vi "Main.vi"() -> ()   [LabVIEW 2019]
doc: "The myRIO Project template acquires acceleration data from the onboard accelerometer and displays the changes of acceleration values in a waveform chart."
uses:
  <vilib>/myRIO/Instrument Drivers/Onboard IO/UART/typedef/VISA Configuration.ctl
  <vilib>/myRIO/Common/Instrument Driver Framework/myRIO v1.0/UART/vis/myRIO v1.0 Close UART.vi
  <vilib>/FPGAPlugInAG/myRIO-1900/niLvFpga_Open_myRIO-1900.vi
  <vilib>/rvi/interface/common/dynamic/niFpgaDynamicAddResources.vi
  <vilib>/Instr/_visa.llb/VISA Configure Serial Port (Instr).vi
  <vilib>/Utility/error.llb/Error Cluster From Error Code.vi
  <vilib>/rvi/errors/niLvFpgaAdjustHostInterfaceError.vi
  <vilib>/myRIO/Common/Instrument Driver Framework/Utilities/vis/FPGA Ref Manager.vi
  <vilib>/myRIO/Common/Instrument Driver Framework/myRIO v1.0/myRIO v1.0 Reset FPGA.vi
  <vilib>/myRIO/Common/Instrument Driver Framework/myRIO v1.0/IRQ/vis/myRIO v1.0 IRQ Info FGV.vi
  <vilib>/myRIO/Common/Instrument Driver Framework/myRIO v1.0/IRQ/vis/myRIO v1.0 Timer IRQ Info FGV.vi
  <vilib>/myRIO/Common/Instrument Driver Framework/myRIO v1.0/IRQ/vis/myRIO v1.0 ISR Agent.vi
  <vilib>/myRIO/Instrument Drivers/Utilities/vis/Reset Index.vi
  <vilib>/myRIO/Common/Instrument Driver Framework/myRIO v1.0/Resource Manager/vis/myRIO v1.0 Block Write Resource Manager.vi
  <vilib>/FPGAPlugInAG/Dynamic/niLvFpga_Close_Dynamic.vi
  <vilib>/rvi/interface/nirviOpenFPGA/nirviOpenFPGA.xnode
  FPGA Bitfiles/PickleRio_FPGATarget_StepperFPGA2.0_025pYRGnFXk.lvbitx
  SubVI/Stepper FPGA 2.0.vi
  <vilib>/myRIO/Express VI/Onboard IO/UART/UART Express VI.xnode
  <vilib>/rvi/interface/nirviReadWriteControl/nirviReadWriteControl.xnode
  <vilib>/rvi/interface/nirviCloseFPGA/nirviCloseFPGA.xnode
  <vilib>/myRIO/Instrument Drivers/Utilities/Utilities.lvlib
  NiFpgaLv.dll
  <vilib>/rvi/interface/Simulation/niFpgaSimulationCallBeginRW.vi
  <vilib>/myRIO/Instrument Drivers/Onboard IO/UART/UART.lvlib
panel:
  in  "KinematicArray":string[](array[string])
  out "Waveform Chart":dynamicdata(graph)
  in  "Speed Robot":dbl
  in  "Stop":bool
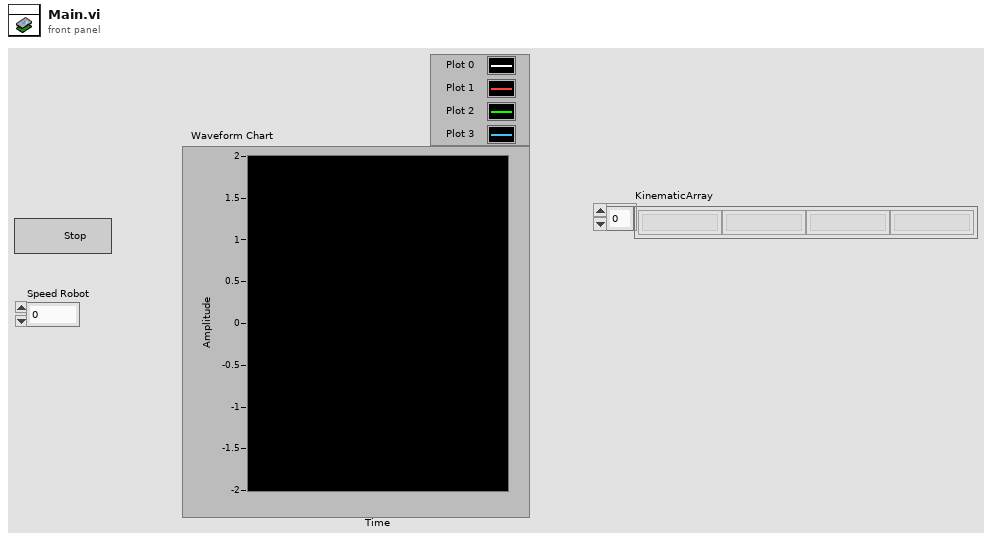
[diagram p1: front panel]
types:
  T1 = cluster{"proportional gain (Kc)":dbl, "integral time (Ti, min)":dbl, "derivative time (Td, min)":dbl}
  T2 = typedef "UART.lvlib/VISA Configuration.ctl" = cluster{"baud rate (9600)":u32, "data bits (8)":u16, "parity (0:none)":enum16{"None", "Odd", "Even", "Mark", "Space"}, "stop bits (10: 1 bit)":u16, "flow control (0:none)":u16, "termination char\n(0xA = '\\n' = LF) ":u8, "Enable Termination\nChar (T)":bool, "timeout (10sec)":u32}
  T3 = cluster{"L1":dbl, "L 2":dbl, "L 3":dbl, " s":dbl, "L1":dbl, "L 2":dbl, "L 3":dbl, " s":dbl}
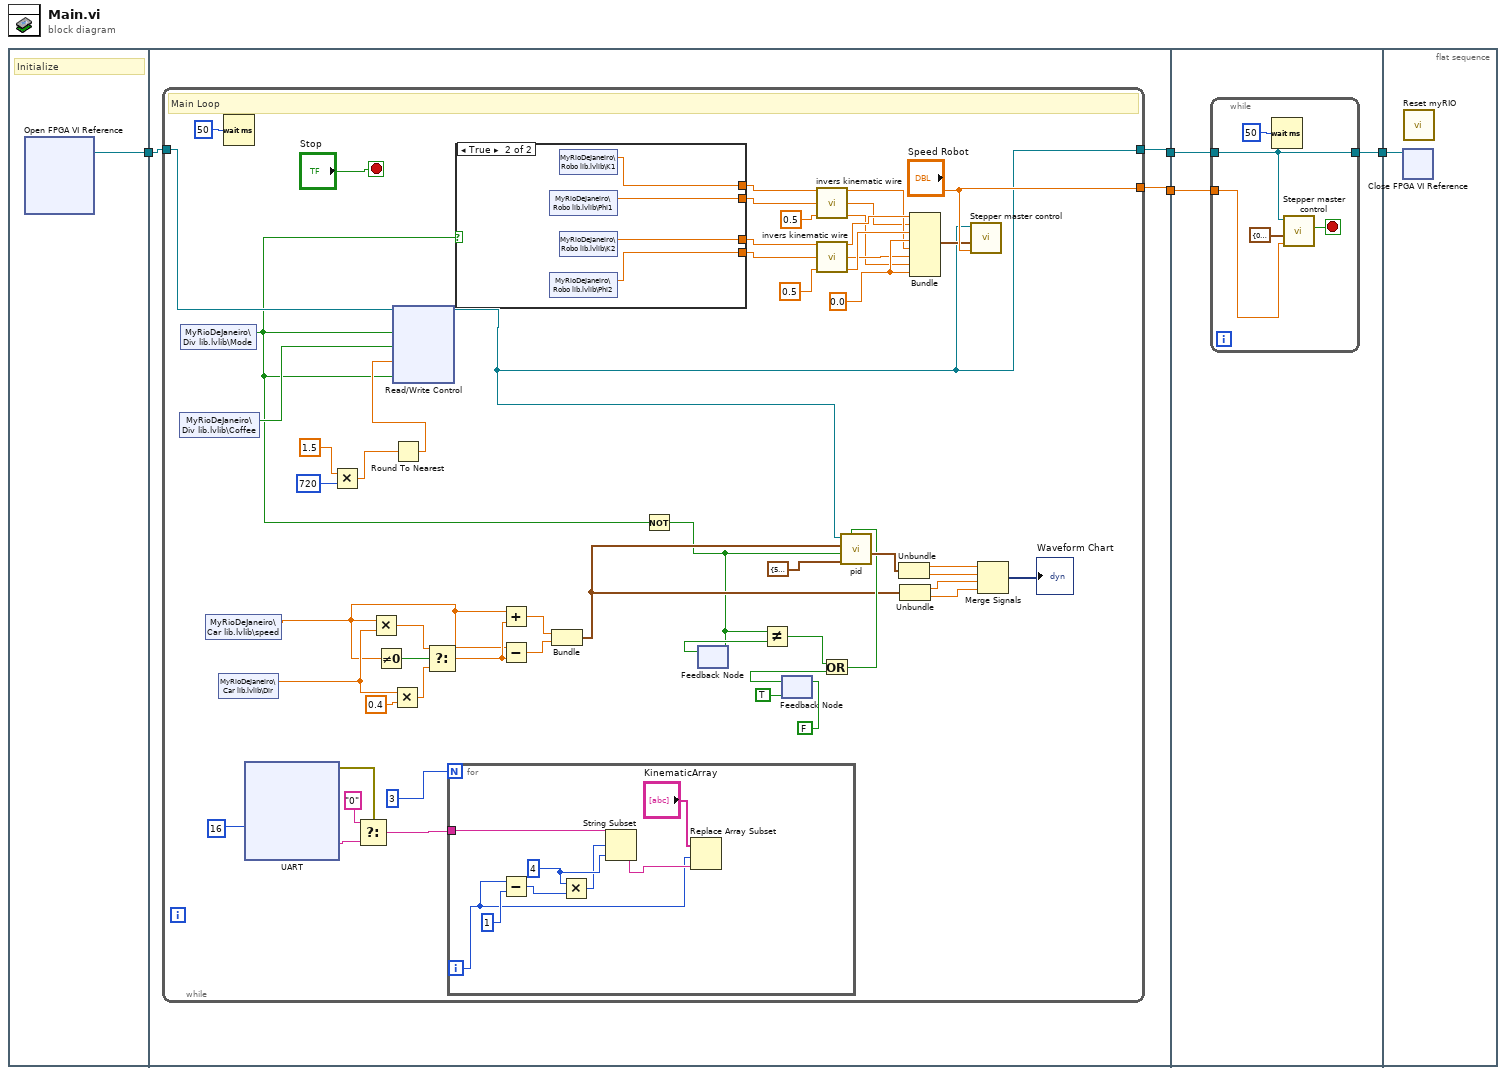
[diagram p0: block diagram]
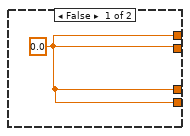
[diagram p2: hidden frame]
diagram:
  n1 = flat-sequence {
    tunnel: [w5] -> w4
    tunnel: w4 -> [w8]
    tunnel: [w7] -> w3
    tunnel: [w6] -> w2
    tunnel: w3 -> [w95]
    tunnel: w2 -> [w94]
    tunnel: [w93] -> w1
    tunnel: w1 -> [w101]
    frame #0 {
      # "Initialize"
      n2 = xnode "Open FPGA VI Reference"() -> ("FPGA VI Reference Out"=w5:refnum<k20>)  [unwired: 2 in, 1 out]
    }
    frame #1 {
      n3 = while {
        tunnel: w8 -> [w45]
        tunnel: ["Speed Robot"] -> w7
        tunnel: [w15] -> w6
        stop <- "Stop" stop-if-true
        w57 = 0.0 ("s")
        # "Main Loop"
        n4 = shared-variable "MyRioDeJaneiro\\Div lib.lvlib\\Coffee"() -> (w21:bool)  [unwired: 1 in, 1 out]
        n5 = shared-variable "MyRioDeJaneiro\\Div lib.lvlib\\Mode"() -> (w17:bool)  [unwired: 1 in, 1 out]
        n6 = shared-variable "MyRioDeJaneiro\\Car lib.lvlib\\speed"() -> (w23:dbl)  [unwired: 1 in, 1 out]
        n7 = shared-variable "MyRioDeJaneiro\\Car lib.lvlib\\Dir"() -> (w24:dbl)  [unwired: 1 in, 1 out]
        n8 = Wait (ms)(milliseconds to wait=u32 50) -> ()  [unwired: 1 out]
        n9 = xnode "UART"("Character Count"=16) -> ("Characters Read"=w13:string, "error out"=w12:errorcluster)  [unwired: 1 in]
        n10 = Multiply(x=1.5, y=i16 720) -> (x*y=w47:dbl)
        n11 = Select(t="0", s=w12, f=w13) -> (s? t:f=w11:string)
        n12 = Multiply(x=w23, y=w24) -> (x*y=w28:dbl)
        n13 = Not Equal To 0?(x=w23) -> (x != 0?=w29:bool)
        n14 = Multiply(x=w24, y=0.4 ("f")) -> (x*y=w26:dbl)
        n15 = Round To Nearest(number=w47) -> (nearest integer value=w46:dbl)
        n16 = xnode "Read/Write Control"("FPGA VI Reference In"=w45, "Pump"=w17, "Coffee"=w21, "cup size"=w46, "Boolean"=w17) -> ("FPGA VI Reference Out"=w15:refnum<k20>)  [unwired: 1 in, 1 out]
        n17 = Select(t=w28, s=w29, f=w26) -> (s? t:f=w27:dbl)
        n18 = for {
          N: 3 -> [_]
          tunnel: w11 -> [w71]
          i -> [w64]
          w68 = 4 ("y")
          n19 = Subtract(x=w64, y=1) -> (x-y=w69:i32)
          n20 = Multiply(x=w68, y=w69) -> (x*y=w67:i32)
          n21 = String Subset(string=w71, offset (0)=w67, length (rest)=w68) -> (substring=w66:string)
          n22 = Replace Array Subset(array="KinematicArray", new element=w66, index=w64) -> ()  [unwired: 1 out]
        }
        n23 = case shown="True" w17 {
          tunnel: [w88 w92] -> w16
          tunnel: [w88 w91] -> w50
          tunnel: [w88 w90] -> w49
          tunnel: [w88 w89] -> w18
          frame False {
            w88 = 0.0
          }
          frame True {
            n24 = shared-variable "MyRioDeJaneiro\\Robo lib.lvlib\\Phi1"() -> (w91:dbl)  [unwired: 1 in, 1 out]
            n25 = shared-variable "MyRioDeJaneiro\\Robo lib.lvlib\\Phi2"() -> (w89:dbl)  [unwired: 1 in, 1 out]
            n26 = shared-variable "MyRioDeJaneiro\\Robo lib.lvlib\\K1"() -> (w92:dbl)  [unwired: 1 in, 1 out]
            n27 = shared-variable "MyRioDeJaneiro\\Robo lib.lvlib\\K2"() -> (w90:dbl)  [unwired: 1 in, 1 out]
          }
        }
        n28 = Add(x=w23, y=w27) -> (x+y=w31:dbl)
        n29 = Subtract(x=w23, y=w27) -> (x-y=w30:dbl)
        n30 = Bundle(w31, w30) -> (w32:cluster{dbl, dbl})  [unwired: 1 in]
        n31 = Not(x=w17) -> (.not. x?=w20:bool)
        n32 = feedback-in #1(w20) -> ()
        n33 = feedback #1() -> (w43:bool)  [unwired: 1 in]
        n34 = Not Equal?(x=w20, y=w43) -> (x != y?=w42:bool)
        n35 = feedback #2(TRUE) -> (w41:bool)
        n36 = feedback-in #2(FALSE) -> ()
        n37 = call "invers kinematic wire.vi"("K"=w16, "phi"=w50, "s"=0.5) -> ("L1"=w53:dbl, "L 2"=w51:dbl, "L 3"=w52:dbl)  [unwired: 10 in]
        n38 = call "invers kinematic wire.vi"("K"=w49, "phi"=w18, "s"=0.5) -> ("L1"=w56:dbl, "L 2"=w54:dbl, "L 3"=w55:dbl)  [unwired: 10 in]
        n39 = Or(x=w42, y=w41) -> (x .or. y?=w33:bool)
        n40 = call "pid.vi"("reset"=w33, "PID gains"=T1 {"proportional gain (Kc)"=53.1, "integral time (Ti, min)"=0.003472, "derivative time (Td, min)"=0.0}, "Enable motors"=w20, "Speed"=w32, "Refnum in"=w15) -> ("output Speed"=w38:cluster{dbl, dbl})  [unwired: 4 in, 2 out]
        n41 = Unbundle(w38) -> (w35:dbl, w34:dbl)
        n42 = Unbundle(w32) -> (w37:dbl, w36:dbl)
        n43 = Bundle("L1"=w56, "L 2"=w51, "L 3"=w55, "s"=w57, "L1"=w53, "L 2"=w54, "L 3"=w52, "s"=w57) -> (w60:T3)  [unwired: 1 in]
        n44 = call "Stepper master control.vi"("Speed"="Speed Robot", "Pos"=w60, "FPGA VI Reference In"=w15) -> ()  [unwired: 8 in, 1 out]
        n45 = Merge Signals(w35, w34, w37, w36) -> (→"Waveform Chart":dynamicdata)
      }
    }
    frame #2 {
      n46 = while {
        tunnel: w95 -> [w99]
        tunnel: w94 -> [w96]
        tunnel: [w96] -> w93
        stop <- w97 stop-if-true
        n47 = Wait (ms)(milliseconds to wait=u32 50) -> ()  [unwired: 1 out]
        n48 = call "Stepper master control.vi"("Speed"=w99, "Pos"=cluster{dbl, dbl, dbl, dbl, dbl, dbl, dbl, dbl} {0.0, 0.0, 0.0, 0.0, 0.0, 0.0, 0.0, 0.0}, "FPGA VI Reference In"=w96) -> ("0?"=w97:bool)  [unwired: 8 in]
      }
    }
    frame #3 {
      n49 = xnode "Close FPGA VI Reference"("FPGA VI Reference In"=w101) -> ()  [unwired: 1 in, 1 out]
      n50 = call <vilib>:"Reset myRIO.vi"() -> ()  [unwired: 11 in, 1 out]
    }
  }
